vi "RH2AH.vi"(1 "RelativeHUmidity":dbl, 2 "Temperature [C]":dbl=243.5) -> (0 "AbsoluteHumidity":dbl)   [LabVIEW 2012]
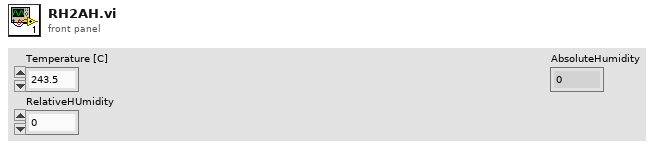
[diagram p1: front panel]
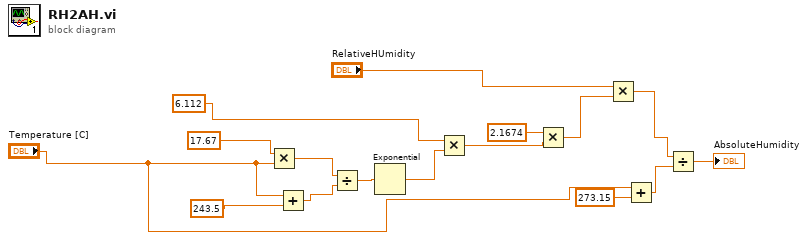
[diagram p0: block diagram]
diagram:
  n1 = Multiply(x=17.67, y="Temperature [C]") -> (x*y=w14:dbl)
  n2 = Add(x="Temperature [C]", y=243.5) -> (x+y=w13:dbl)
  n3 = Divide(x=w14, y=w13) -> (x/y=w12:dbl)
  n4 = Exponential(1:w12) -> (0:w10:dbl)
  n5 = Multiply(x=6.112, y=w10) -> (x*y=w9:dbl)
  n6 = Multiply(x=2.1674, y=w9) -> (x*y=w4:dbl)
  n7 = Multiply(x="RelativeHUmidity", y=w4) -> (x*y=w3:dbl)
  n8 = Add(x="Temperature [C]", y=273.15) -> (x+y=w5:dbl)
  n9 = Divide(x=w3, y=w5) -> (x/y=→"AbsoluteHumidity":dbl)
